vi "RMDestroyAll.vi"() -> ()   [LabVIEW 2011]
uses:
  QTrkDLL.vi
panel:
  out "error":errorcluster
  in  "error in (no error)":errorcluster
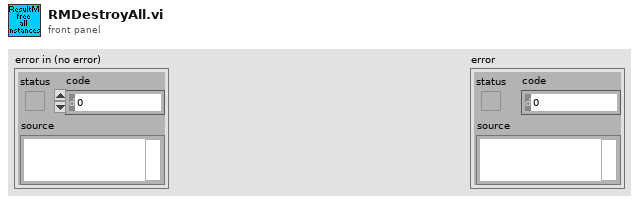
[diagram p1: front panel]
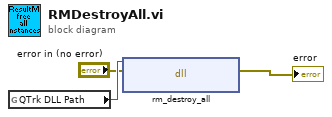
[diagram p0: block diagram]
diagram:
  n1 = global read "QTrkDLL.vi" "QTrk DLL Path"() -> (w3:path)
  n2 = dll-call lib="D:/jcnossen1/cudaqi-tracker/bin/jtrk-labview.dll" fn="rm_destroy_all"(path in=w3, error in="error in (no error)") -> (error out=→"error":errorcluster)  [unwired: 2 in, 1 out]
